vi "FTW-JSON-LexicalScan-IntegerDeserialize.vi"(7 "Byte Array":u8[](array[numeric])) -> (8 "Variant":variant)   [LabVIEW 2015]
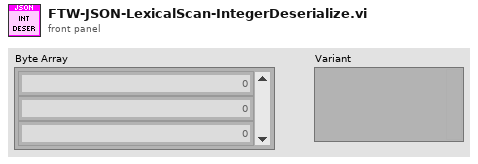
[diagram p1: front panel]
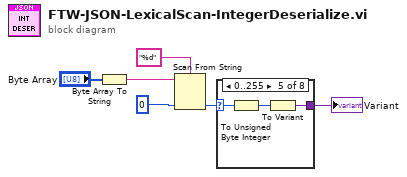
[diagram p0: block diagram]
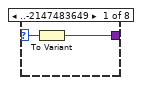
[diagram p2: hidden frame]
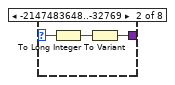
[diagram p3: hidden frame]
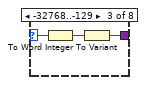
[diagram p4: hidden frame]
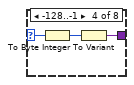
[diagram p5: hidden frame]
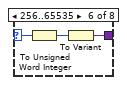
[diagram p6: hidden frame]
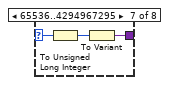
[diagram p7: hidden frame]
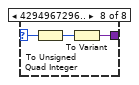
[diagram p8: hidden frame]
diagram:
  n1 = Byte Array To String(unsigned byte array="Byte Array") -> (string=w3:string)
  n2 = Scan From String(format string="%d", input string=w3, default 1=i64 0) -> (output 1=w5:i64)  [unwired: 2 in, 3 out]
  n3 = case shown="0..255" w5 {
    selector: w5 -> [w8 w11 w14 w17 w20 w23 w26 w29]
    tunnel: [w7 w10 w13 w16 w19 w22 w25 w28] -> w6
    frame ..-2147483649 {
      n4 = To Variant(anything=w8) -> (Variant=w7:variant)
    }
    frame -2147483648..-32769 {
      n5 = To Long Integer(number=w11) -> (32bit integer=w9:i32)
      n6 = To Variant(anything=w9) -> (Variant=w10:variant)
    }
    frame -32768..-129 {
      n7 = To Word Integer(number=w14) -> (16bit integer=w12:i16)
      n8 = To Variant(anything=w12) -> (Variant=w13:variant)
    }
    frame -128..-1 {
      n9 = To Byte Integer(number=w17) -> (8bit integer=w15:i8)
      n10 = To Variant(anything=w15) -> (Variant=w16:variant)
    }
    frame 0..255 {
      n11 = To Unsigned Byte Integer(number=w20) -> (unsigned 8bit integer=w18:u8)
      n12 = To Variant(anything=w18) -> (Variant=w19:variant)
    }
    frame 256..65535 {
      n13 = To Unsigned Word Integer(number=w23) -> (unsigned 16bit integer=w21:u16)
      n14 = To Variant(anything=w21) -> (Variant=w22:variant)
    }
    frame 65536..4294967295 {
      n15 = To Unsigned Long Integer(number=w26) -> (unsigned 32bit integer=w24:u32)
      n16 = To Variant(anything=w24) -> (Variant=w25:variant)
    }
    frame 4294967296.. {
      n17 = To Unsigned Quad Integer(1:w29) -> (0:w27:u64)
      n18 = To Variant(anything=w27) -> (Variant=w28:variant)
    }
  }
  "Variant" <- w6
